vi "Test Quantum Design.vi"() -> ()   [LabVIEW 2018]
uses:
  Quantum Design Driver/Quantum Desing Configuration.ctl
  Quantum Design Driver/Quantum Design Driver.lvclass
panel:
  out "Waveform Chart":dbl[][](graph)
  in  "Stop Button":bool
  in  "Update period":dbl=1.0 format="%#_6ps"
  in  "Quantum Desing Configuration":T1={"Address"="127.0.0.1", "Instrument type"=0, "Remote"=TRUE, "Temperature"=TRUE, "Field"=TRUE} {"Instrument type" items=["PPMS", "VersaLab", "DynaCool", "SVSM"]}
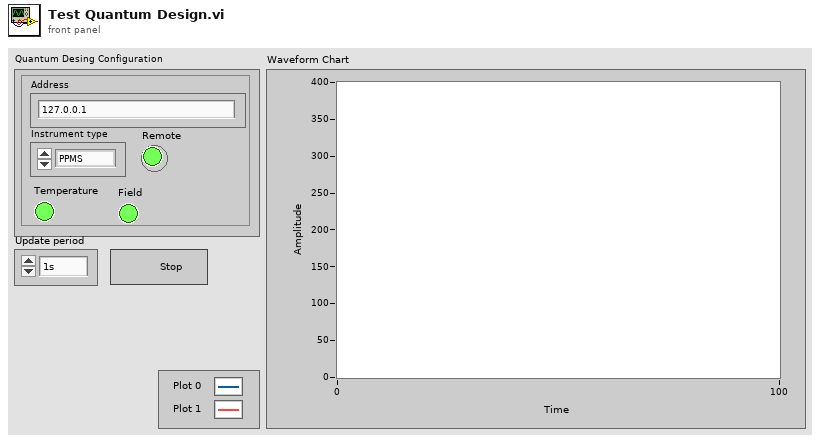
[diagram p1: front panel]
types:
  T1 = typedef "Quantum Desing Configuration.ctl" = cluster{"Address":string, "Instrument type":u16, "Remote":bool, "Temperature":bool, "Field":bool}
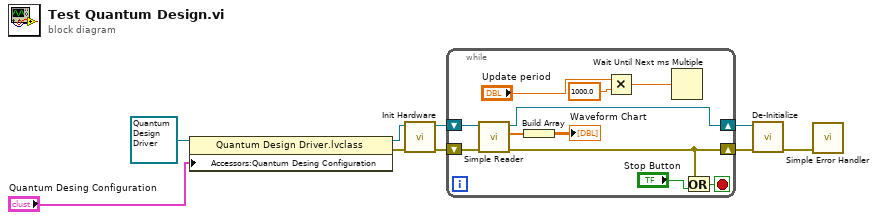
[diagram p0: block diagram]
diagram:
  n1 = property class="Quantum Design Driver.lvclass"(reference=refnum<class "Quantum Design Driver.lvclass"> refnum ("Quantum Design Driver.lvclass"), "Accessors:Quantum Desing Configuration"="Quantum Desing Configuration") -> (reference out=w8:refnum<class "Quantum Design Driver.lvclass">, error out=w6:errorcluster)  [unwired: 1 in]
  n2 = call-dynamic "Init Hardware.vi"("error in (no error)"=w6, "Quantum Design Driver in"=w8) -> ("error out"=w5:errorcluster, "Quantum Design Driver out"=w4:refnum<class "Quantum Design Driver.lvclass">)  [unwired: 8 in]
  n3 = while {
    shift-right: [w11] -> w2
    shift-left: w5 -> [w19]
    shift-right: [w18] -> w3
    shift-left: w4 -> [w20]
    stop <- w13 stop-if-true
    n4 = call-dynamic "Simple Reader.vi"("error in (no error)"=w19, "Quantum Design Driver in"=w20) -> ("error out"=w11:errorcluster, "Signals"=w14:dbl[], "Quantum Design Driver out"=w18:refnum<class "Quantum Design Driver.lvclass">)  [unwired: 7 in]
    n5 = Build Array(w14) -> (→"Waveform Chart":dbl[][])
    n6 = Multiply(x="Update period", y=1000.0) -> (x*y=w16:dbl)
    n7 = Wait Until Next ms Multiple(millisecond multiple=w16) -> ()  [unwired: 1 out]
    n8 = Or(x=w11, y="Stop Button") -> (x .or. y?=w13:bool)
  }
  n9 = call-dynamic "De-Initialize.vi"("error in (no error)"=w2, "Quantum Design Driver in"=w3) -> ("error out"=w1:errorcluster)  [unwired: 8 in, 1 out]
  n10 = call <vilib>:"Simple Error Handler.vi"("error in (no error)"=w1) -> ()  [unwired: 4 in, 5 out]
